vi "MagnetorotGUI.vi"() -> ()   [LabVIEW 2016]
uses:
  <vilib>/Instr/_visa.llb/VISA Configure Serial Port (Instr).vi
panel:
  in  "Raw Write":bool
  out "Write String":string
  in  "Set RPM":bool
  in  "RPM":dbl=60.0
  in  "stop":bool
  in  "Set Speed":bool
  in  "Speed":dbl=1570.0
  out "Output":string
  out "Write LED":bool
  out "Error":errorcluster
  in  "Raw String":string="help\n"
  out "read string":string
  in  "VISA resource name":refnum<visa-resource-name>="COM1"
  in  "baud rate":u32=115200
  out "Pulse":i64
  in  "Quit":bool
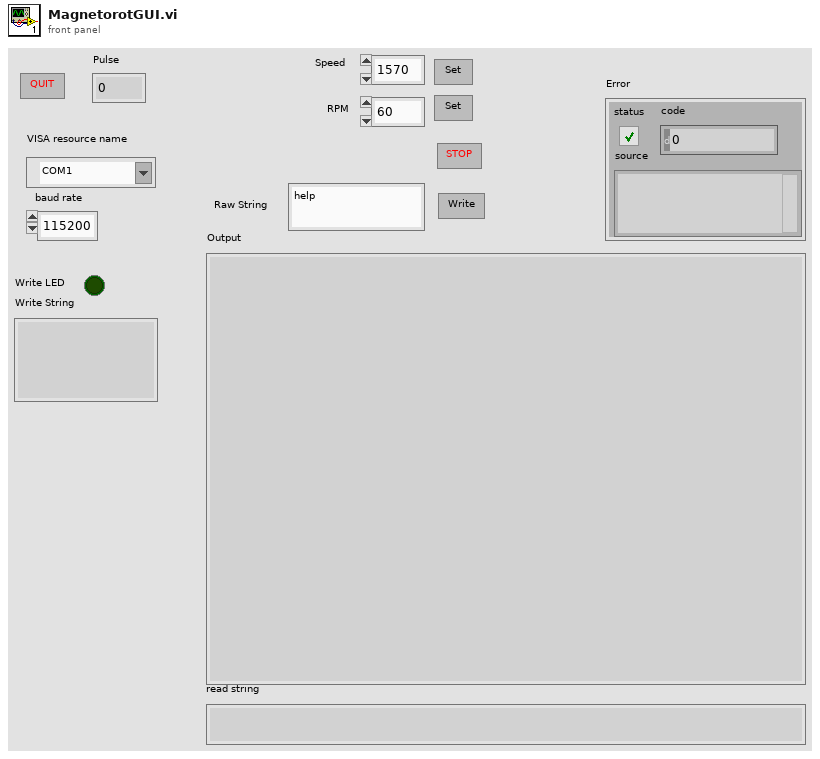
[diagram p1: front panel]
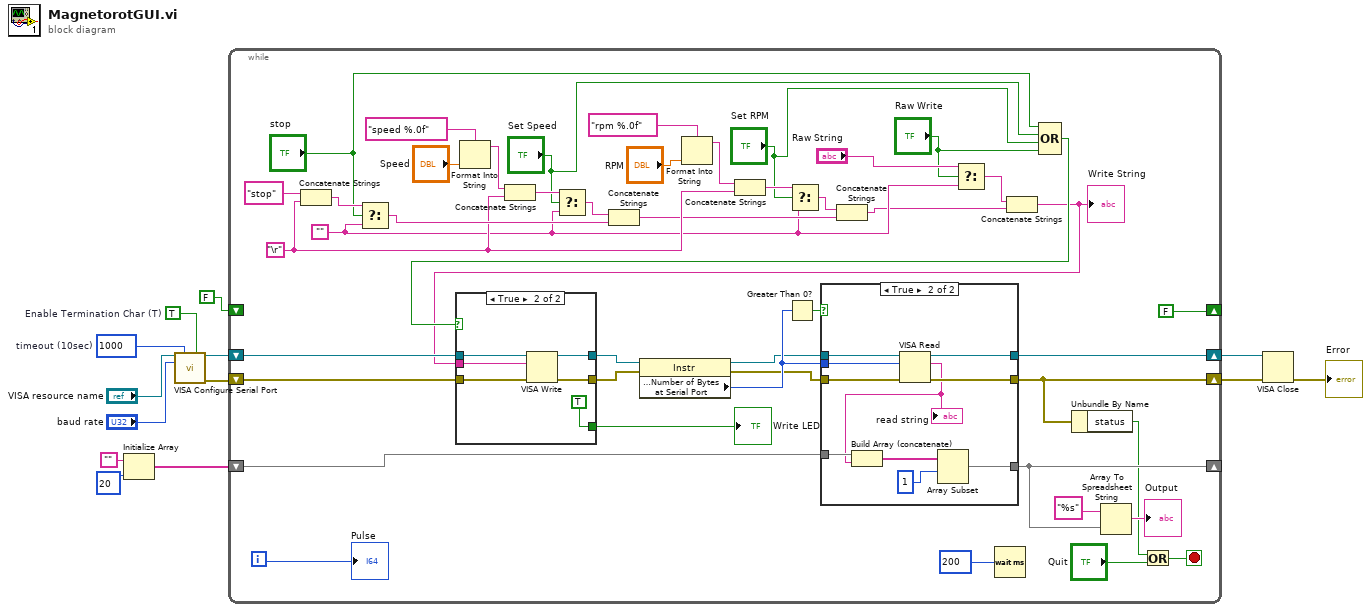
[diagram p0: block diagram]
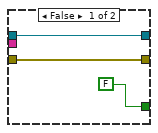
[diagram p3: hidden frame]
diagram:
  w9 = TRUE  # Enable Termination Char (T)
  w10 = u32 1000  # timeout (10sec)
  n1 = Initialize Array("", 20) -> (w1:string[])
  n2 = call-poly "VISA Configure Serial Port"("VISA resource name"="VISA resource name", "timeout (10sec)"=w10, "Enable Termination\nChar (T)"=w9, "baud rate (9600)"="baud rate") -> ("VISA resource name out"=w13:refnum<visa-resource-name>, "error out"=w5:errorcluster)  [unwired: 10 in]
  n3 = while {
    shift-right: [w56] -> w12
    shift-left: w13 -> [w50]
    shift-right: [FALSE] -> _
    shift-left: FALSE -> [_]
    shift-right: [w55] -> w6
    shift-left: w5 -> [w49]
    shift-right: [w43] -> _
    shift-left: w1 -> [w44]
    i -> [w39]
    stop <- w54 stop-if-true
    w26 = "\r"
    w22 = ""
    n4 = Concatenate Strings("stop", w26) -> (w34:string)
    n5 = Select(t=w34, s="stop", f=w22) -> (s? t:f=w30:string)
    n6 = Format Into String(format string="speed %.0f", "Speed") -> (resulting string=w32:string)  [unwired: 2 in, 1 out]
    n7 = Concatenate Strings(w32, w26) -> (w33:string)
    n8 = Select(t=w33, s="Set Speed", f=w22) -> (s? t:f=w31:string)
    n9 = Concatenate Strings(w31, w30) -> (w24:string)
    n10 = Format Into String(format string="rpm %.0f", "RPM") -> (resulting string=w25:string)  [unwired: 2 in, 1 out]
    n11 = Concatenate Strings(w25, w26) -> (w29:string)
    n12 = Select(t=w29, s="Set RPM", f=w22) -> (s? t:f=w28:string)
    n13 = Concatenate Strings(w28, w24) -> (w20:string)
    n14 = Select(t="Raw String", s="Raw Write", f=w22) -> (s? t:f=w21:string)
    n15 = Wait (ms)(milliseconds to wait=200) -> ()  [unwired: 1 out]
    n16 = Concatenate Strings(w21, w20) -> (w14:string)
    "Write String" <- w14
    n17 = Compound Arithmetic op=OR("stop", "Set Speed", "Set RPM", "Raw Write") -> (w15:bool)
    n18 = case shown="True" w15 {
      tunnel: w50 -> [w75 w81]
      tunnel: [w75 w80] -> w48
      tunnel: [FALSE TRUE] -> w58
      tunnel: w49 -> [w73 w78]
      tunnel: [w73 w77] -> w46
      tunnel: w14 -> [_ w76]
      frame False {
      }
      frame True {
        n19 = VISA Write(VISA resource name=w81, write buffer=w76, error in (no error)=w78) -> (VISA resource name out=w80:refnum<visa-resource-name>, error out=w77:errorcluster)  [unwired: 1 out]
      }
    }
    "Write LED" <- w58
    n20 = property class="Instr"(reference=w48, error in=w46) -> (reference out=w47:refnum<visa-resource-name>, error out=w45:errorcluster, "Serial Settings:Number of Bytes at Serial Port"=w51:u32)
    n21 = Greater Than 0?(x=w51) -> (x > 0?=w52:bool)
    n22 = case shown="True" w52 {
      tunnel: w47 -> [w62 w72]
      tunnel: w45 -> [w61 w71]
      tunnel: [w61 w70] -> w55
      tunnel: [w62 w69] -> w56
      tunnel: w51 -> [_ w68]
      tunnel: w44 -> [w60 w67]
      tunnel: [w60 w65] -> w43
      frame False {
      }
      frame True {
        n23 = VISA Read(VISA resource name=w72, byte count=w68, error in (no error)=w71) -> (VISA resource name out=w69:refnum<visa-resource-name>, read buffer=w64:string, error out=w70:errorcluster)  [unwired: 1 out]
        "read string" <- w64
        n24 = Build Array (concatenate)(w67, w64) -> (w66:string[])
        n25 = Array Subset(array=w66, index=1) -> (w65:string[])  [unwired: 1 in]
      }
    }
    n26 = Unbundle By Name(w55) -> ("status"=w40:bool)
    n27 = Array To Spreadsheet String(array=w43, 3:"%s") -> (spreadsheet string=→"Output":string)  [unwired: 1 in]
    n28 = Or(x=w40, y="Quit") -> (x .or. y?=w54:bool)
    "Pulse" <- w39
  }
  n29 = VISA Close(VISA resource name=w12, error in (no error)=w6) -> (error out=→"Error":errorcluster)
